vi "Write Status.vi"(8 "error in (no error)":errorcluster, 10 "Status":string, 11 "Caraya Status Data in":refnum<class "Caraya Status Data.lvclass">) -> (0 "error out":errorcluster, 3 "Caraya Status Data out":refnum<class "Caraya Status Data.lvclass">)   [LabVIEW 2019, in "ProjectBuilder.lvlib" / "Caraya Status Data.lvclass"]
doc: "Write the status string to the private data."
uses:
  Caraya Status Data.lvclass
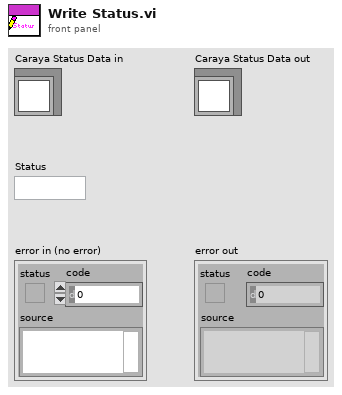
[diagram p1: front panel]
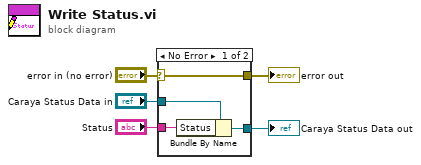
[diagram p0: block diagram]
diagram:
  n1 = case shown="No Error" "error in (no error)" {
    selector: "error in (no error)" -> [w9 w10]
    tunnel: [w9 w10] -> w4
    tunnel: [w7 w11] -> w2
    tunnel: "Caraya Status Data in" -> [w8 w11]
    tunnel: "Status" -> [w6 _]
    frame No Error {
      n2 = Bundle By Name(cluster=w8, "Status"=w6) -> (w7:refnum<class "Caraya Status Data.lvclass">)
    }
    frame Error {
    }
  }
  "error out" <- w4
  "Caraya Status Data out" <- w2
